vi "getfiresettings.vi"(8 "error in (no error)":errorcluster, 11 "hObject":i32=1) -> (0 "error out":errorcluster, 2 "pSettings":T1, 3 "hObject Out":i32=1)   [LabVIEW 2009]
doc: "This vi finds the available compatible devices on the network.\n\n<B>DeviceType</B>: device to find. multiple device types can be used by using the <B>logical OR</B> operator\n\n<B>Error In</B> : If error, then this call will be skipped and the error is passed through\n\n<B>NeoDevices {}</B> : the found devices array\n\n<B>pNumDevices</B> : number of devices found\n\n<B>Error Out</B> : returns the error produced by the call\n\n12/21/2010 1.0.0 jyg\n- initial release"
uses:
  ctl firesetting.ctl
  NEO VI Example/data/icsneo40.dll
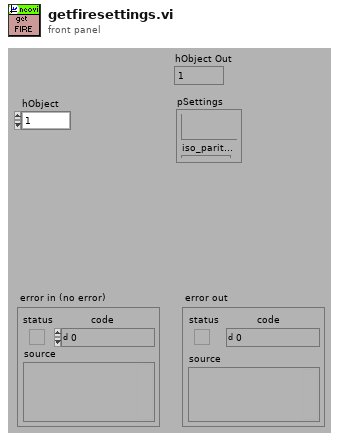
[diagram p1: front panel]
types:
  T1 = typedef "ctl FireSetting.ctl" = cluster{"can 1":cluster{"Mode":u8, "SetBaudrate":u8, "Baudrate":u8, "NetworkType":u8, "TqSeg1":u8, "TqSeg2":u8, "TqProp":u8, "TqSync":u8, "BRP":u16, "auto_baud":u16}, "can 2":cluster{"Mode":u8, "SetBaudrate":u8, "Baudrate":u8, "NetworkType":u8, "TqSeg1":u8, "TqSeg2":u8, "TqProp":u8, "TqSync":u8, "BRP":u16, "auto_baud":u16}, "can 3":cluster{"Mode":u8, "SetBaudrate":u8, "Baudrate":u8, "NetworkType":u8, "TqSeg1":u8, "TqSeg2":u8, "TqProp":u8, "TqSync":u8, "BRP":u16, "auto_baud":u16}, "can 4":cluster{"Mode":u8, "SetBaudrate":u8, "Baudrate":u8, "NetworkType":u8, "TqSeg1":u8, "TqSeg2":u8, "TqProp":u8, "TqSync":u8, "BRP":u16, "auto_baud":u16}, "swcan":cluster{"Mode":u8, "SetBaudrate":u8, "Baudrate":u8, "NetworkType":u8, "TqSeg1":u8, "TqSeg2":u8, "TqProp":u8, "TqSync":u8, "BRP":u16, "high_speed_auto_switch":u16, "auto_baud":u16}, "lsftcan":cluster{"Mode":u8, "SetBaudrate":u8, "Baudrate":u8, "NetworkType":u8, "TqSeg1":u8, "TqSeg2":u8, "TqProp":u8, "TqSync":u8, "BRP":u16, "auto_baud":u16}, "lin 1":cluster{"Baudrate":u32, "spbrg":u16, "brgh":u16, "MasterResistor":u8, "Mode":u8}, "lin 2":cluster{"Baudrate":u32, "spbrg":u16, "brgh":u16, "MasterResistor":u8, "Mode":u8}, "lin 3":cluster{"Baudrate":u32, "spbrg":u16, "brgh":u16, "MasterResistor":u8, "Mode":u8}, "lin 4":cluster{"Baudrate":u32, "spbrg":u16, "brgh":u16, "MasterResistor":u8, "Mode":u8}, "cgi_enable":u16, "cgi_baud":u16, "cgi_tx_ifs_bit_times":u16, "cgi_rx_ifs_bit_times":u16, "cgi_chksum_enable":u16, "network_enalbes":u16, "network_enabled_on_boot":u16, "pwm_man_timeout":u16, "pwm_man_enable":u16, "misc_io_initial_ddr":u16, "misc_io_initial_latch":u16, "misc_io_analog_enable":u16, "misc_io_report_period":u16, "misc_io_on_report_events":u16, "ain_sample_period":u16, "ain_threshold":u16, "iso15765_separation_time_offset":u16, "iso9141_kwp_enable":u16, "ISO9141_Settings":cluster{"Baudrate":u32, "spbrg":u16, "brgh":u16, "ISO9141_KEYWORD2000_INIT_STEP":cluster{"time_500us":u16, "k":u16, "l":u16}, "init_step_count":u8, "p2_500us":u16, "p3_500us":u16, "p4_500us":u16, "chksum_enabled":u16}, "perf_en":u16, "iso_parity":u16, "iso_msg_termination":u16, "iso_tester_pullup_enable":u16, "network_enables_2":u16, "ISO9141__Settings2":cluster{"Baudrate":u32, "spbrg":u16, "brgh":u16, "ISO9141_KEYWORD2000_INIT_STEP":cluster{"time_500us":u16, "k":u16, "l":u16}, "init_step_count":u8, "p2_500us":u16, "p3_500us":u16, "p4_500us":u16, "chksum_enabled":u16}, "iso_parity_2":u16, "iso_msg_termination_2":u16, "ISO9141_Settings_3":cluster{"Baudrate":u32, "spbrg":u16, "brgh":u16, "ISO9141_KEYWORD2000_INIT_STEP":cluster{"time_500us":u16, "k":u16, "l":u16}, "init_step_count":u8, "p2_500us":u16, "p3_500us":u16, "p4_500us":u16, "chksum_enabled":u16}, "iso_parity_3":u16, "iso_msg_termination_3":u16, "ISO9141_Settings_4":cluster{"Baudrate":u32, "spbrg":u16, "brgh":u16, "ISO9141_KEYWORD2000_INIT_STEP":cluster{"time_500us":u16, "k":u16, "l":u16}, "init_step_count":u8, "p2_500us":u16, "p3_500us":u16, "p4_500us":u16, "chksum_enabled":u16}, "iso_parity_4":u16, "iso_msg_termination_4":u16}
  T2 = cluster{"can 1":cluster{"Mode":u8, "SetBaudrate":u8, "Baudrate":u8, "NetworkType":u8, "TqSeg1":u8, "TqSeg2":u8, "TqProp":u8, "TqSync":u8, "BRP":u16, "auto_baud":u16}, "can 2":cluster{"Mode":u8, "SetBaudrate":u8, "Baudrate":u8, "NetworkType":u8, "TqSeg1":u8, "TqSeg2":u8, "TqProp":u8, "TqSync":u8, "BRP":u16, "auto_baud":u16}, "can 3":cluster{"Mode":u8, "SetBaudrate":u8, "Baudrate":u8, "NetworkType":u8, "TqSeg1":u8, "TqSeg2":u8, "TqProp":u8, "TqSync":u8, "BRP":u16, "auto_baud":u16}, "can 4":cluster{"Mode":u8, "SetBaudrate":u8, "Baudrate":u8, "NetworkType":u8, "TqSeg1":u8, "TqSeg2":u8, "TqProp":u8, "TqSync":u8, "BRP":u16, "auto_baud":u16}, "swcan":cluster{"Mode":u8, "SetBaudrate":u8, "Baudrate":u8, "NetworkType":u8, "TqSeg1":u8, "TqSeg2":u8, "TqProp":u8, "TqSync":u8, "BRP":u16, "high_speed_auto_switch":u16, "auto_baud":u16}, "lsftcan":cluster{"Mode":u8, "SetBaudrate":u8, "Baudrate":u8, "NetworkType":u8, "TqSeg1":u8, "TqSeg2":u8, "TqProp":u8, "TqSync":u8, "BRP":u16, "auto_baud":u16}, "lin 1":cluster{"Baudrate":u32, "spbrg":u16, "brgh":u16, "MasterResistor":u8, "Mode":u8}, "lin 2":cluster{"Baudrate":u32, "spbrg":u16, "brgh":u16, "MasterResistor":u8, "Mode":u8}, "lin 3":cluster{"Baudrate":u32, "spbrg":u16, "brgh":u16, "MasterResistor":u8, "Mode":u8}, "lin 4":cluster{"Baudrate":u32, "spbrg":u16, "brgh":u16, "MasterResistor":u8, "Mode":u8}, "cgi_enable":u16, "cgi_baud":u16, "cgi_tx_ifs_bit_times":u16, "cgi_rx_ifs_bit_times":u16, "cgi_chksum_enable":u16, "network_enalbes":u16, "network_enabled_on_boot":u16, "pwm_man_timeout":u16, "pwm_man_enable":u16, "misc_io_initial_ddr":u16, "misc_io_initial_latch":u16, "misc_io_analog_enable":u16, "misc_io_report_period":u16, "misc_io_on_report_events":u16, "ain_sample_period":u16, "ain_threshold":u16, "iso15765_separation_time_offset":u16, "iso9141_kwp_enable":u16, "ISO9141_Settings":cluster{"Baudrate":u32, "spbrg":u16, "brgh":u16, "ISO9141_KEYWORD2000_INIT_STEP":cluster{"time_500us":u16, "k":u16, "l":u16}, "init_step_count":u8, "p2_500us":u16, "p3_500us":u16, "p4_500us":u16, "chksum_enabled":u16}, "perf_en":u16, "iso_parity":u16, "iso_msg_termination":u16, "iso_tester_pullup_enable":u16, "network_enables_2":u16, "ISO9141__Settings2":cluster{"Baudrate":u32, "spbrg":u16, "brgh":u16, "ISO9141_KEYWORD2000_INIT_STEP":cluster{"time_500us":u16, "k":u16, "l":u16}, "init_step_count":u8, "p2_500us":u16, "p3_500us":u16, "p4_500us":u16, "chksum_enabled":u16}, "iso_parity_2":u16, "iso_msg_termination_2":u16, "ISO9141_Settings_3":cluster{"Baudrate":u32, "spbrg":u16, "brgh":u16, "ISO9141_KEYWORD2000_INIT_STEP":cluster{"time_500us":u16, "k":u16, "l":u16}, "init_step_count":u8, "p2_500us":u16, "p3_500us":u16, "p4_500us":u16, "chksum_enabled":u16}, "iso_parity_3":u16, "iso_msg_termination_3":u16, "ISO9141_Settings_4":cluster{"Baudrate":u32, "spbrg":u16, "brgh":u16, "ISO9141_KEYWORD2000_INIT_STEP":cluster{"time_500us":u16, "k":u16, "l":u16}, "init_step_count":u8, "p2_500us":u16, "p3_500us":u16, "p4_500us":u16, "chksum_enabled":u16}, "iso_parity_4":u16, "iso_msg_termination_4":u16}
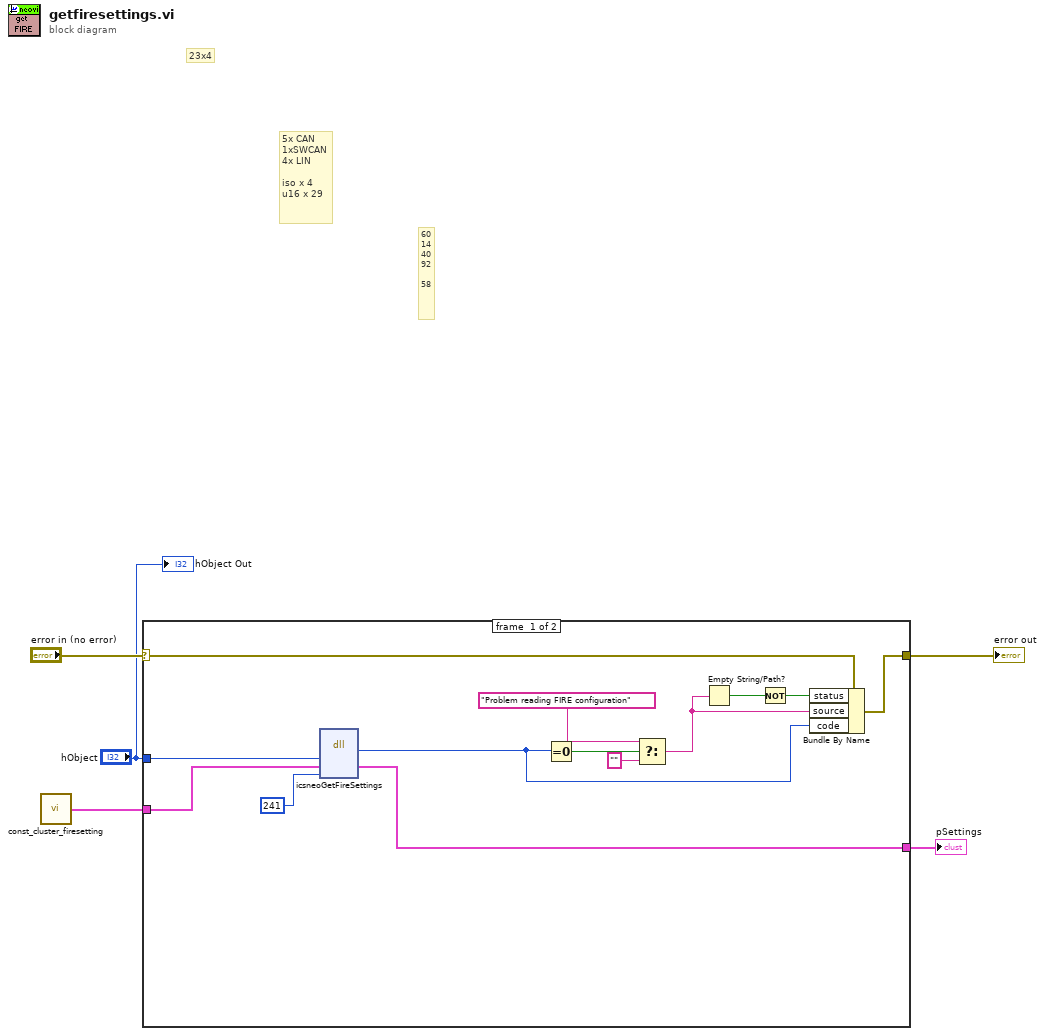
[diagram p0: block diagram]
diagram:
  # "23x4"
  # "60\n14\n40\n92\n\n58"
  # "5x CAN\n1xSWCAN\n4x LIN\n\niso x 4\nu16 x 29"
  n1 = call "const_cluster_firesetting.vi"() -> ("firesetting {}"=w2:T2)
  n2 = case shown="No Error" "error in (no error)" {
    selector: "error in (no error)" -> [w14 w19]
    tunnel: [w15 w19] -> w5
    tunnel: "hObject" -> [w10 _]
    tunnel: w2 -> [w9 _]
    tunnel: [w7 _] -> w1
    frame #0 {
      n3 = dll-call lib="C:/WINDOWS/system32/icsneo40.dll" fn="icsneoGetFireSettings"("hObject"=w10, "pSettings"=w9, "iNumBytes"=241) -> ("return type"=w13:i32, "pSettings"=w7:T2)  [unwired: 5 in, 2 out]
      n4 = Equal To 0?(x=w13) -> (x = 0?=w12:bool)
      n5 = Select(t="Problem reading FIRE configuration", s=w12, f="") -> (s? t:f=w11:string)
      n6 = Empty String/Path?(string/path=w11) -> (empty?=w17:bool)
      n7 = Not(x=w17) -> (.not. x?=w16:bool)
      n8 = Bundle By Name(cluster=w14, "status"=w16, "source"=w11, "code"=w13) -> (w15:errorcluster)
    }
    frame #1 {
    }
  }
  "error out" <- w5
  "pSettings" <- w1
  "hObject Out" <- "hObject"
